vi "GetDataEventBlockInfo.vi"(8 "operating state properties":T1[](array[typedef]), 9 "group properties":T1[](array[typedef]), 10 "channels":T2[](array[typedef]), 11 "default data block length":dbl) -> (0 "type":T4, 1 "pritrigger":i32, 2 "total length":dbl, 3 "speed reference":string, 4 "enter pretrigger":i32, 6 "enter total length":dbl)   [LabVIEW 2017, in "DataAccumulator.lvlib"]
uses:
  <vilib>/addons/InsightCM/Devices/Shared/Common/DataAccumulator/DataAccumulator.lvlib
  <vilib>/addons/InsightCM/Devices/Shared/Common/DataAccumulator/controls/accumulationType.ctl
  <vilib>/addons/InsightCM/MessageBus/Base/controls/KeyValuePair.ctl
  <vilib>/addons/InsightCM/MessageBus/Base/controls/R2_Channel.ctl
  <vilib>/addons/InsightCM/MessageBus/Base/controls/Metric.ctl
  <vilib>/addons/InsightCM/Utilities/PropertyHelpers/PropertyHelpers.lvlib
  <vilib>/addons/InsightCM/Utilities/DeviceModelHelpers/DeviceModelHelpers.lvlib
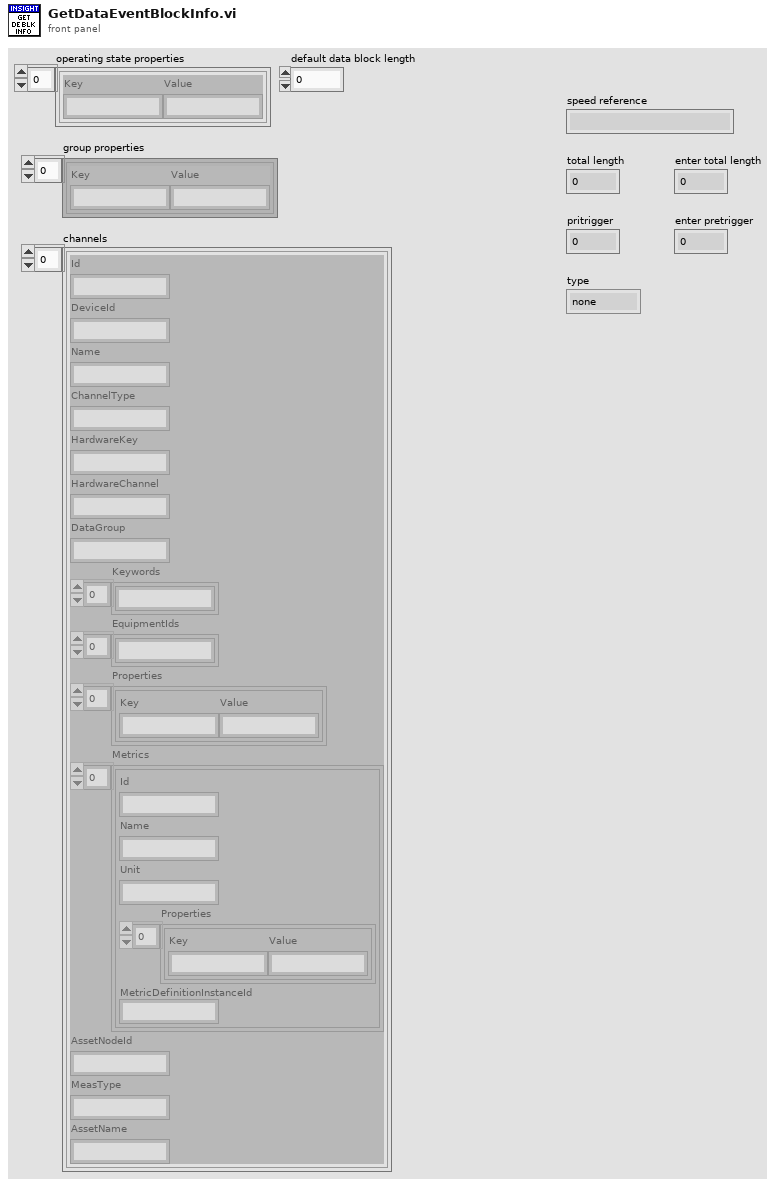
[diagram p1: front panel]
types:
  T1 = typedef "KeyValuePair.ctl" = cluster{"Key":string, "Value":string}
  T2 = typedef "R2_Channel.ctl" = cluster{"Id":string, "DeviceId":string, "Name":string, "ChannelType":string, "HardwareKey":string, "HardwareChannel":string, "DataGroup":string, "Keywords":string[], "EquipmentIds":string[], "Properties":T1[], "Metrics":T3[], "AssetNodeId":string, "MeasType":string, "AssetName":string}
  T3 = typedef "Metric.ctl" = cluster{"Id":string, "Name":string, "Unit":string, "Properties":T1[], "MetricDefinitionInstanceId":string}
  T4 = typedef "DataAccumulator.lvlib/accumulationType.ctl" = enum16{"none", "seconds", "revolutions"}
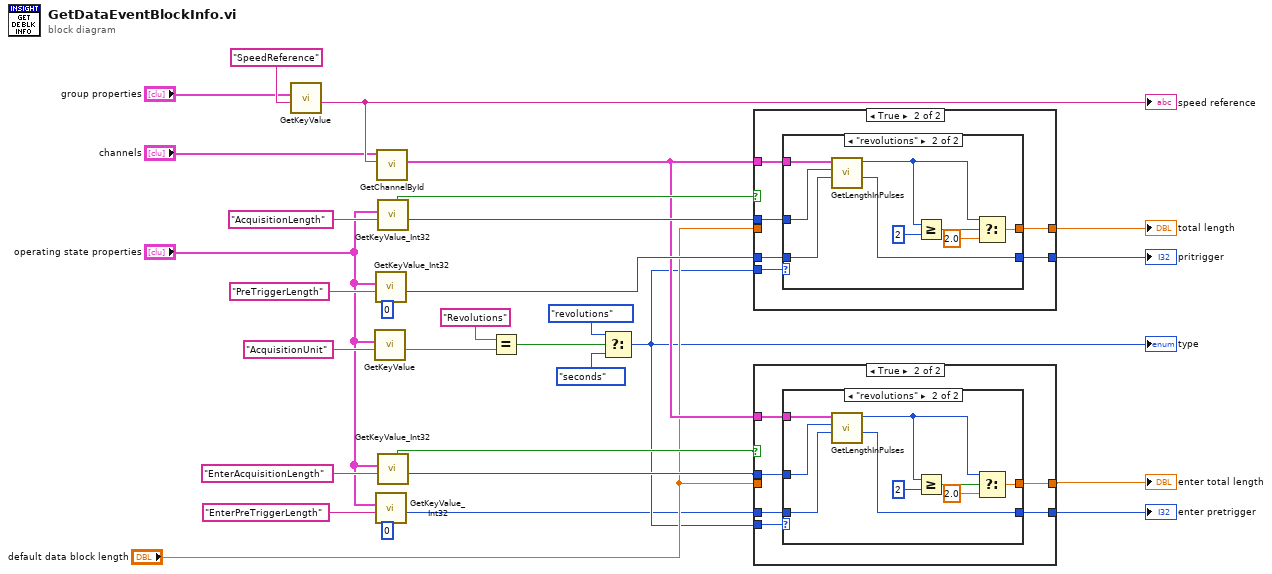
[diagram p0: block diagram]
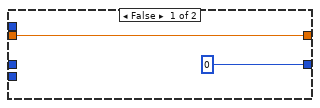
[diagram p2: hidden frame]
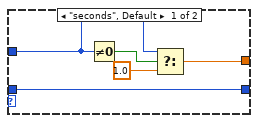
[diagram p3: hidden frame]
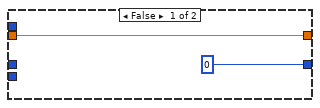
[diagram p4: hidden frame]
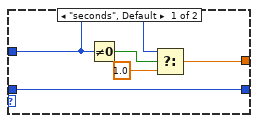
[diagram p5: hidden frame]
diagram:
  n1 = call <vilib>:"GetKeyValue.vi"("key"="SpeedReference", "key value pairs"="group properties") -> ("value"=w26:string)  [unwired: 7 in, 2 out]
  "speed reference" <- w26
  n2 = call <vilib>:"GetKeyValue.vi"("key"="AcquisitionUnit", "key value pairs"="operating state properties") -> ("value"=w19:string)  [unwired: 7 in, 2 out]
  n3 = call <vilib>:"GetKeyValue_Int32.vi"("default"=0, "key"="PreTriggerLength", "key value pairs"="operating state properties") -> ("value"=w13:i32)  [unwired: 6 in, 2 out]
  n4 = call <vilib>:"GetKeyValue_Int32.vi"("default"=0, "key"="EnterPreTriggerLength", "key value pairs"="operating state properties") -> ("value"=w3:i32)  [unwired: 6 in, 2 out]
  n5 = call <vilib>:"GetChannelById.vi"("channel id"=w26, "channels in"="channels") -> ("channel"=w8:T2)  [unwired: 7 in, 2 out]
  n6 = call <vilib>:"GetKeyValue_Int32.vi"("key"="AcquisitionLength", "key value pairs"="operating state properties") -> ("value"=w14:i32, "found"=w12:bool)  [unwired: 7 in, 1 out]
  n7 = call <vilib>:"GetKeyValue_Int32.vi"("key"="EnterAcquisitionLength", "key value pairs"="operating state properties") -> ("value"=w6:i32, "found"=w7:bool)  [unwired: 7 in, 1 out]
  n8 = Equal?(x="Revolutions", y=w19) -> (x = y?=w9:bool)
  n9 = Select(t=accumulationType."revolutions" ("Accumulation Settings.Type"), s=w9, f=accumulationType."seconds" ("Accumulation Settings.Type")) -> (s? t:f=w4:T4)
  "type" <- w4
  n10 = case shown="True" w12 {
    tunnel: w8 -> [_ w38]
    tunnel: [0 ("value") w37] -> w10
    tunnel: w14 -> [_ w36]
    tunnel: w13 -> [_ w35]
    tunnel: [w31 w34] -> w11
    tunnel: "default data block length" -> [w31 _]
    tunnel: w4 -> [_ w33]
    frame False {
    }
    frame True {
      n11 = case shown="\"revolutions\"" w33 {
        tunnel: w38 -> [_ w51]
        tunnel: [w39 w47] -> w37
        tunnel: w36 -> [w40 w50]
        tunnel: w35 -> [w39 w49]
        tunnel: [w41 w48] -> w34
        frame "seconds", Default {
          n12 = Not Equal To 0?(x=w40) -> (x != 0?=w43:bool)
          n13 = Select(t=w40, s=w43, f=1.0) -> (s? t:f=w41:dbl)
        }
        frame "revolutions" {
          n14 = call <vilib>:"GetLengthInPulses.vi"("pretrig"=w49, "revolutions"=w50, "speed ref channel"=w51) -> ("pretrigger length in pulses"=w47:i32, "total length in pulses"=w46:i32)  [unwired: 6 in, 1 out]
          n15 = Greater Or Equal?(x=w46, y=2) -> (x >= y?=w44:bool)
          n16 = Select(t=w46, s=w44, f=2.0) -> (s? t:f=w48:dbl)
        }
      }
    }
  }
  "pritrigger" <- w10
  "total length" <- w11
  n17 = case shown="True" w7 {
    tunnel: w8 -> [_ w60]
    tunnel: [0 ("value") w59] -> w1
    tunnel: w6 -> [_ w58]
    tunnel: w3 -> [_ w57]
    tunnel: [w53 w56] -> w2
    tunnel: "default data block length" -> [w53 _]
    tunnel: w4 -> [_ w55]
    frame False {
    }
    frame True {
      n18 = case shown="\"revolutions\"" w55 {
        tunnel: w60 -> [_ w73]
        tunnel: [w61 w69] -> w59
        tunnel: w58 -> [w62 w72]
        tunnel: w57 -> [w61 w71]
        tunnel: [w63 w70] -> w56
        frame "seconds", Default {
          n19 = Not Equal To 0?(x=w62) -> (x != 0?=w65:bool)
          n20 = Select(t=w62, s=w65, f=1.0) -> (s? t:f=w63:dbl)
        }
        frame "revolutions" {
          n21 = call <vilib>:"GetLengthInPulses.vi"("pretrig"=w71, "revolutions"=w72, "speed ref channel"=w73) -> ("pretrigger length in pulses"=w69:i32, "total length in pulses"=w68:i32)  [unwired: 6 in, 1 out]
          n22 = Greater Or Equal?(x=w68, y=2) -> (x >= y?=w66:bool)
          n23 = Select(t=w68, s=w66, f=2.0) -> (s? t:f=w70:dbl)
        }
      }
    }
  }
  "enter total length" <- w2
  "enter pretrigger" <- w1
